vi "Write Fetch Room Details Msg.vi"(10 "Guest Manager UI.lvlib:Fetch Room Details Msg.lvclass":refnum<class "Fetch Room Details Msg.lvclass">, 11 "Guest Manager UI in":refnum<class "Guest Manager UI.lvclass">) -> (3 "Guest Manager UI out":refnum<class "Guest Manager UI.lvclass">)   [LabVIEW 2023, in "Guest Manager UI.lvlib" / "Guest Manager UI.lvclass"]
uses:
  Guest Manager UI.lvclass
  Guest Manager UI Messages/Fetch Room Details Msg/Fetch Room Details Msg.lvclass
  Guest Manager UI.lvclass/Guest Manager UI.ctl
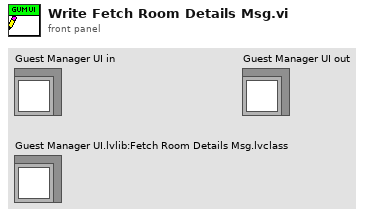
[diagram p1: front panel]
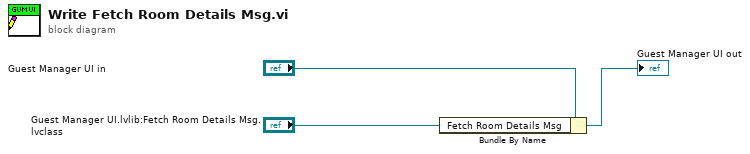
[diagram p0: block diagram]
diagram:
  n1 = Bundle By Name(cluster="Guest Manager UI in", "Fetch Room Details Msg"="Guest Manager UI.lvlib:Fetch Room Details Msg.lvclass") -> (→"Guest Manager UI out":refnum<class "Guest Manager UI.lvclass">)
